vi "lp-server.vi"() -> ()   [LabVIEW 2019]
uses:
  vi.lib/addons/zeromq/socket_type.ctl
  vi.lib/addons/zeromq/zmq_context.lvclass
  vi.lib/addons/zeromq/zeromq.lvlib
  vi.lib/addons/zeromq/zmq_socket.lvclass
panel:
  in  "stop?":bool
  out "loop":i32
  in  "endpoint":string="tcp://127.0.0.1:5555"
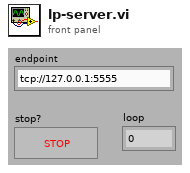
[diagram p1: front panel]
types:
  T1 = typedef "zeromq.lvlib/socket_type.ctl" = enum8{"ZMQ_PAIR", "ZMQ_PUB", "ZMQ_SUB", "ZMQ_REQ", "ZMQ_REP", "ZMQ_DEALER", "ZMQ_ROUTER", "ZMQ_PULL", "ZMQ_PUSH", "ZMQ_XPUB", "ZMQ_XSUB"}
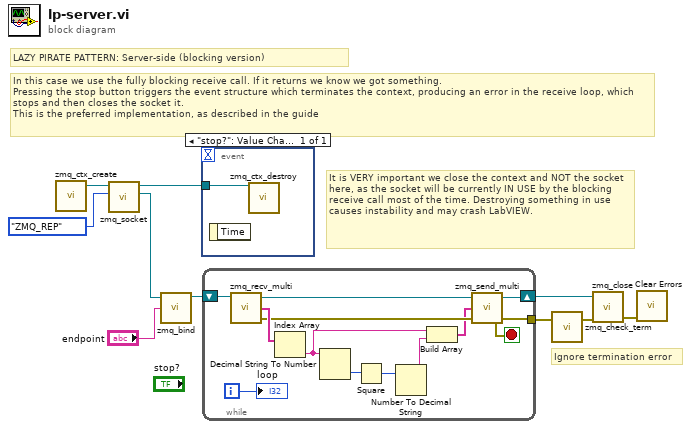
[diagram p0: block diagram]
diagram:
  # "Ignore termination error"
  # "It is VERY important we close the context and NOT the socket here, as the socket will be currently IN USE by the blocking receive call most of the time. Destroying something in use causes instability and may crash LabVIEW."
  # "In this case we use the fully blocking receive call. If it returns we know we got something.\nPressing the stop button triggers the event structure which terminates the context, producing an error in the receive loop, which stops and then closes the socket it.\nThis is the preferred implementation, as described in the guide"
  # "LAZY PIRATE PATTERN: Server-side (blocking version)"
  n1 = call "zmq_ctx_create.vi"() -> ("context out"=w6:refnum<class "zmq_context.lvclass">)  [unwired: 4 in, 1 out]
  n2 = call "zmq_socket.vi"("socket type"=socket_type."ZMQ_REP", "context in"=w6) -> ("socket out"=w5:refnum<class "zmq_socket.lvclass">, "context out"=w4:refnum<class "zmq_context.lvclass">)  [unwired: 3 in, 1 out]
  n3 = call "zmq_bind.vi"("endpoint"="endpoint", "socket in"=w5) -> ("socket out"=w9:refnum<class "zmq_socket.lvclass">)  [unwired: 2 in, 1 out]
  n4 = event shown="[0] \"stop?\": Value Change" {
    selector: _ -> [_]
    dyn-events: _ -> [_]
    timeout: _ -> [_]
    tunnel: w4 -> [w11]
    event "stop?": Value Change {
      n5 = event-data() -> ()  [unwired: 1 in, 1 out]
      n6 = call "zmq_ctx_destroy.vi"("context in"=w11) -> ()  [unwired: 4 in, 1 out]
    }
  }
  n7 = while {
    shift-right: [w18] -> w7
    shift-left: w9 -> [w23]
    tunnel: [w15] -> w2
    i -> [w17]
    stop <- w15 stop-if-true
    n8 = call "zmq_recv_multi.vi"("socket in"=w23) -> ("error out"=w16:errorcluster, "parts"=w21:string[], "socket out"=w22:refnum<class "zmq_socket.lvclass">)  [unwired: 2 in]
    n9 = Index Array(array=w21) -> (element=w14:string)  [unwired: 1 in]
    n10 = Decimal String To Number(string=w14) -> (number=w20:i32)  [unwired: 2 in, 1 out]
    n11 = Square(x=w20) -> (x^2=w19:i32)
    n12 = Number To Decimal String(number=w19) -> (decimal integer string=w13:string)  [unwired: 1 in]
    n13 = Build Array(w14, w13) -> (w12:string[])
    n14 = call "zmq_send_multi.vi"("error in"=w16, "parts"=w12, "socket in"=w22) -> ("error out"=w15:errorcluster, "socket out"=w18:refnum<class "zmq_socket.lvclass">)  [unwired: 1 in]
    "loop" <- w17
  }
  n15 = call "zmq_check_term.vi"("error in"=w2) -> ("error out"=w1:errorcluster)  [unwired: 1 in, 1 out]
  n16 = call "zmq_close.vi"("error in"=w1, "socket"=w7) -> ("error out"=w3:errorcluster)  [unwired: 3 in]
  n17 = call <vilib>:"Clear Errors.vi"("error in (no error)"=w3) -> ()  [unwired: 5 in, 2 out]
